vi "Acknowledge Post Process.vi"(8 "error in (no error)":errorcluster, 9 "Open plot":bool, 10 "Ack Result":refnum<class "Acquired Result.lvclass">, 11 "Monitor-Pulse in":refnum<class "Application Controller.lvclass">) -> (0 "error out":errorcluster, 2 "Complete":bool, 3 "Monitor-Pulse out":refnum<class "Application Controller.lvclass">)   [LabVIEW 2016, in "Application Controller.lvclass"]
uses:
  Application Controller.lvclass
  NHMFL_Core/Libraries/Instruments/Results/Acquired Result/Acquired Result.lvclass
  Process Object Messages/Process Result Msg/Process Result Msg.lvclass/Process Result Msg.ctl
  <vilib>/ActorFramework/Message Enqueuer/Message Enqueuer.lvclass/Message Enqueuer.ctl
  <vilib>/ActorFramework/Message Enqueuer/Enqueue.vi
  Process Object Messages/Process Result Msg/Process Result Msg.lvclass
  C:/Program Files/National Instruments/LabVIEW 2016/vi.lib/ActorFramework/Message/Message.lvclass
  <vilib>/ActorFramework/Message Priority Queue/Priority Enqueue.vi
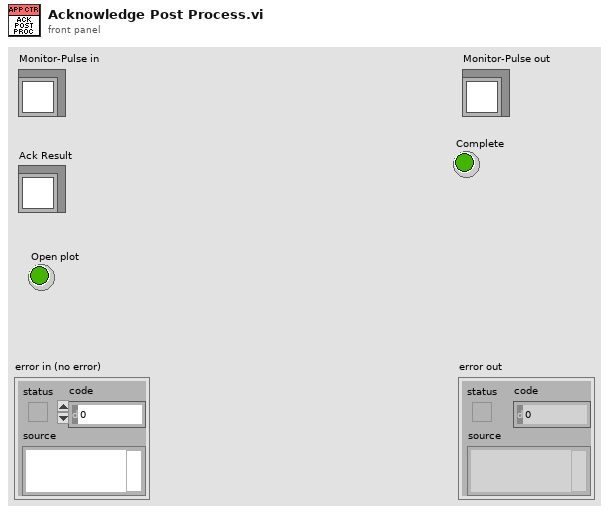
[diagram p1: front panel]
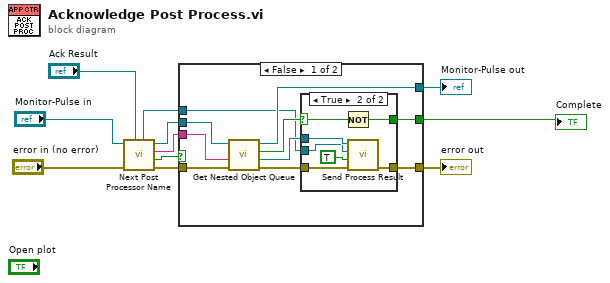
[diagram p0: block diagram]
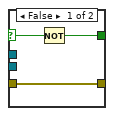
[diagram p2: hidden frame]
diagram:
  n1 = call-dynamic "Next Post Processor Name.vi"("Ack Result"="Ack Result", "error in (no error)"="error in (no error)", "Monitor-Pulse in"="Monitor-Pulse in") -> ("error out"=w6:errorcluster, "Complete"=w4:bool, "Post processor name"=w8:string, "Monitor-Pulse out"=w9:refnum<class "Application Controller.lvclass">, "Ack Result out"=w2:refnum<class "Acquired Result.lvclass">)  [unwired: 4 in]
  n2 = case shown="False" w4 {
    selector: w4 -> [_ w32]
    tunnel: w9 -> [w21 w33]
    tunnel: w8 -> [w20 _]
    tunnel: [w16 w33] -> w7
    tunnel: w6 -> [w15 w34]
    tunnel: [w14 w34] -> w5
    tunnel: w2 -> [w13 _]
    tunnel: [w12 w32] -> w1
    frame False {
      n3 = call-dynamic "Get Nested Object Queue.vi"("error in (no error)"=w15, "Name"=w20, "Measure Object in"=w21) -> ("error out"=w18:errorcluster, "Object Enqueuer"=w17:refnum<class "Message Enqueuer.lvclass">, "Found?"=w19:bool, "Measure Object out"=w16:refnum<class "Application Controller.lvclass">)  [unwired: 5 in]
      n4 = case shown="True" w19 {
        selector: w19 -> [w23 w26]
        tunnel: w17 -> [_ w31]
        tunnel: w18 -> [w24 w30]
        tunnel: [w24 w29] -> w14
        tunnel: w13 -> [_ w28]
        tunnel: [w22 w25] -> w12
        frame False {
          n5 = Not(x=w23) -> (.not. x?=w22:bool)
        }
        frame True {
          n6 = Not(x=w26) -> (.not. x?=w25:bool)
          n7 = call "Send Process Result.vi"("error in (no error)"=w30, "Acknowledge"=TRUE, "Result in"=w28, "Message Enqueuer"=w31) -> ("error out"=w29:errorcluster)  [unwired: 6 in, 1 out]
        }
      }
    }
    frame True {
    }
  }
  "error out" <- w5
  "Monitor-Pulse out" <- w7
  "Complete" <- w1
